vi "Sr830 AuxOut.vi"(4 "error in":errorcluster, 5 "AuxOut Ch":u16(ring)=1 items=["1"=1, "2"=2, "3"=3, "4"=4], 6 "Voltage":dbl min=-10.5 max=10.5 step=0.001, 7 "Ressource VISA":refnum<visa-resource-name>="GPIB0::8::INSTR") -> (0 "error out":errorcluster, 2 "Voltage Out":dbl min=-10.5 max=10.5 step=0.001, 3 "Ressource VISA Out":refnum<visa-resource-name>="GPIB0::8::INSTR")   [LabVIEW 2019]
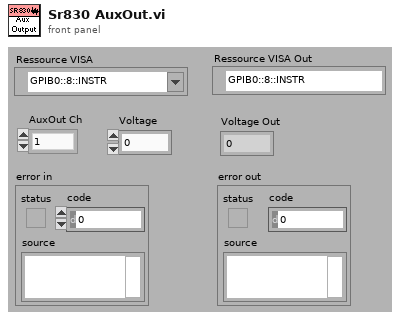
[diagram p1: front panel]
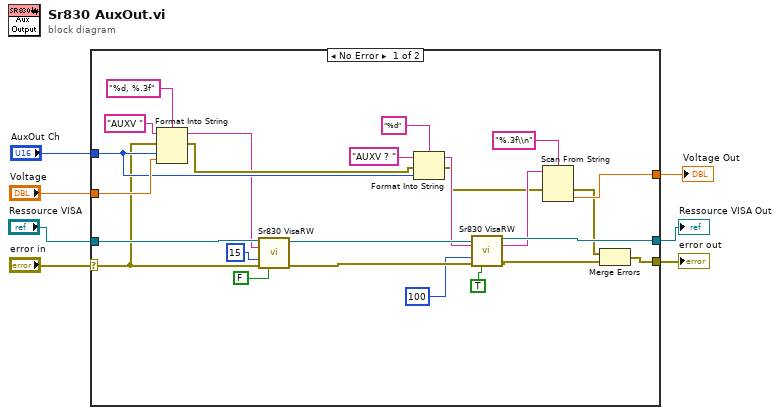
[diagram p0: block diagram]
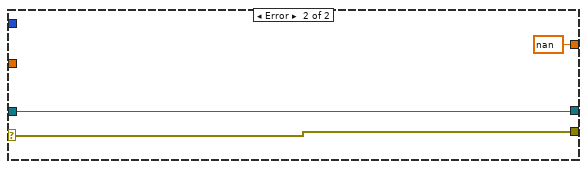
[diagram p2: hidden frame]
diagram:
  n1 = case shown="No Error" "error in" {
    selector: "error in" -> [w18 w35]
    tunnel: [w9 w35] -> w7
    tunnel: "Ressource VISA" -> [w31 w34]
    tunnel: [w27 w34] -> w4
    tunnel: "AuxOut Ch" -> [w24 _]
    tunnel: "Voltage" -> [w25 _]
    tunnel: [w12 nan] -> w1
    frame No Error {
      n2 = Format Into String(format string="%d, %.3f" ("chaîne de format"), initial string="AUXV " ("ChaineCom"), error in=w18, w24, w25) -> (resulting string=w16:string, error out=w17:errorcluster)
      n3 = call <userlib>:"Sr830 VisaRW.vi"("VISA Rsrc"=w31, "ChaineCom"=w16, "Nbcaract"=u32 15, "error in (no error)"=w18, "Lecture?(T)"=FALSE) -> ("VISA Rsrc Out"=w28:refnum<visa-resource-name>, "error out"=w29:errorcluster)  [unwired: 7 in, 2 out]
      n4 = Format Into String(format string="%d" ("chaîne de format"), initial string="AUXV ? " ("ChaineCom"), error in=w17, w24) -> (resulting string=w20:string, error out=w10:errorcluster)
      n5 = call <userlib>:"Sr830 VisaRW.vi"("VISA Rsrc"=w28, "ChaineCom"=w20, "Nbcaract"=u32 100, "error in (no error)"=w29, "Lecture?(T)"=TRUE) -> ("VISA Rsrc Out"=w27:refnum<visa-resource-name>, "ChaineRep"=w14:string, "error out"=w11:errorcluster)  [unwired: 7 in, 1 out]
      n6 = Scan From String(format string="%.3f\\n", input string=w14, error in=w10) -> (error out=w8:errorcluster, output 1=w12:dbl)  [unwired: 2 in, 2 out]
      n7 = Merge Errors(w8, w11) -> (w9:errorcluster)
    }
    frame Error {
    }
  }
  "error out" <- w7
  "Ressource VISA Out" <- w4
  "Voltage Out" <- w1
